vi "Parse Datagram.vi"(4 "source address":u32, 6 "source port":u16, 7 "transfer group id":i32, 8 "error in (no error)":errorcluster, 10 "datagram":string, 11 "UDP Transceiver in":refnum<class "UDP Transceiver.lvclass">=refnum) -> (0 "error out":errorcluster, 1 "valid":bool, 2 "transfer data":string, 3 "UDP Transceiver out":refnum<class "UDP Transceiver.lvclass">, 5 "transfer id":i32)   [LabVIEW 2020, in "UDP.lvlib" / "UDP Transceiver.lvclass"]
uses:
  UDP Transceiver.lvclass
  Throw Unknown Datagram Error.vi
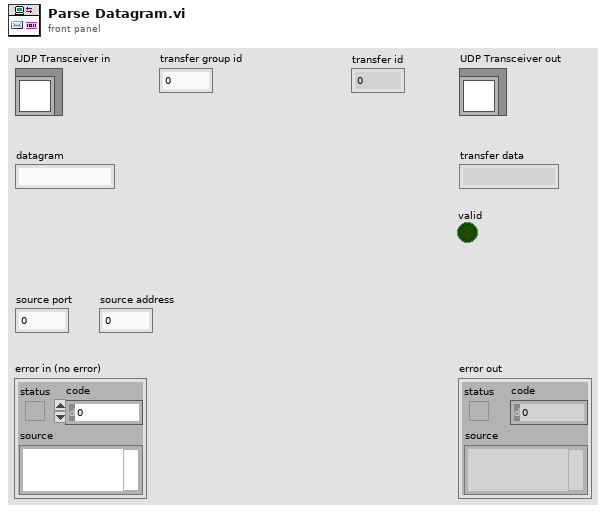
[diagram p1: front panel]
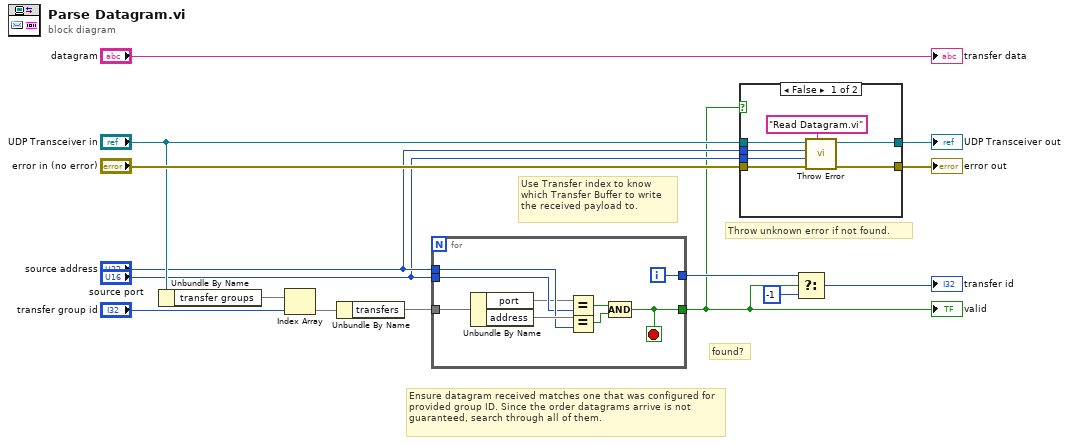
[diagram p0: block diagram]
diagram:
  # "Throw unknown error if not found."
  # "Use Transfer index to know which Transfer Buffer to write the received payload to."
  # "found?"
  # "Ensure datagram received matches one that was configured for provided group ID. Since the order datagrams arrive is not guaranteed, search through all of them."
  n1 = Unbundle By Name("UDP Transceiver in") -> ("transfer groups"=w10)
  n2 = Index Array(array=w10, index="transfer group id") -> (element=w8)
  n3 = Unbundle By Name(w8) -> ("transfers"=w15)
  n4 = for {
    tunnel: w15 -> [w20]
    tunnel: [w22] -> w3
    tunnel: [w21] -> w2
    tunnel: "source port" -> [w17]
    tunnel: "source address" -> [w18]
    i -> [w22]
    stop <- w21 stop-if-true
    n5 = Unbundle By Name(w20) -> ("port"=w16, "address"=w19)
    n6 = Equal?(x=w16, y=w17) -> (x = y?=w23:bool)
    n7 = Equal?(x=w19, y=w18) -> (x = y?=w24:bool)
    n8 = Compound Arithmetic op=AND(w23, w24) -> (w21:bool)
  }
  "valid" <- w2
  n9 = case shown="False" w2 {
    tunnel: "error in (no error)" -> [w30 w32]
    tunnel: "UDP Transceiver in" -> [w31 w33]
    tunnel: [w29 w33] -> w14
    tunnel: [w28 w32] -> w13
    tunnel: "source port" -> [w26 _]
    tunnel: "source address" -> [w25 _]
    frame False {
      n10 = call-poly "Throw Error.vi"("source vi name"="Read Datagram.vi", "error in (no error)"=w30, "source port"=w26, "source address"=w25, "UDP in"=w31) -> ("error out"=w28:errorcluster, "UDP out"=w29:refnum<class "UDP Transceiver.lvclass">)  [unwired: 5 in]
    }
    frame True {
    }
  }
  "error out" <- w13
  "UDP Transceiver out" <- w14
  n11 = Select(t=w3, s=w2, f=-1) -> (s? t:f=→"transfer id":i32)
  "transfer data" <- "datagram"
